vi "Arduino-Open.vi"(6 "Max number timeouts":u32=20, 7 "Enable Termination\nChar (T)":bool=TRUE, 8 "error in (no error)":errorcluster, 9 "termination char\n(0xA = '\\n' = LF)":u8=10 format="%.0x", 10 "baud rate (9600)":u32=9600, 11 "Visa Resource":refnum<visa-resource-name>) -> (0 "error out":errorcluster, 2 "Moin, moin!":string, 3 "VISA resource name out":refnum<visa-resource-name>)   [LabVIEW 2018]
uses:
  <vilib>/Instr/_visa.llb/VISA Configure Serial Port (Instr).vi
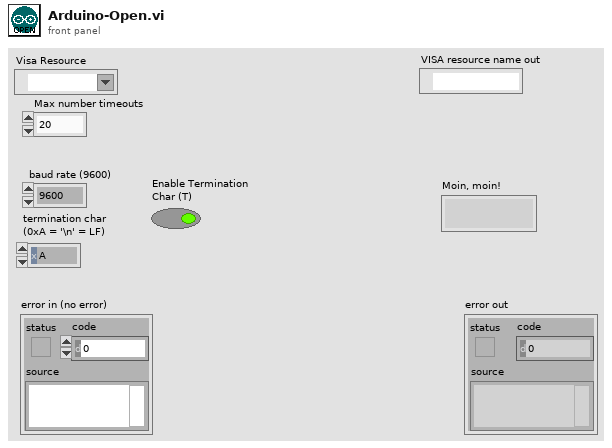
[diagram p1: front panel]
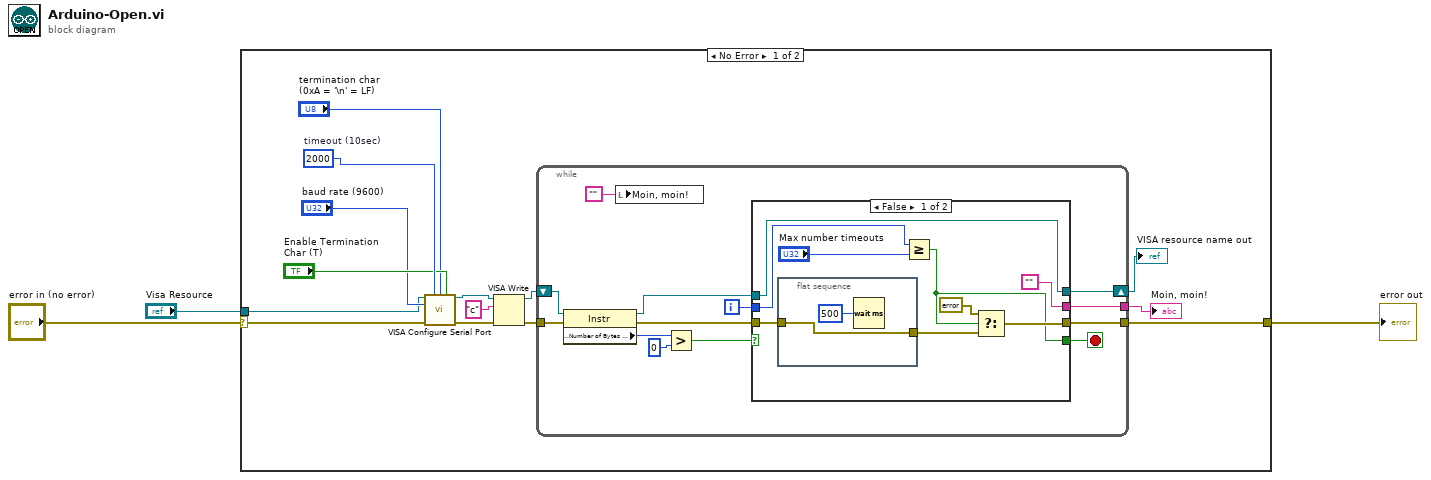
[diagram p0: block diagram]
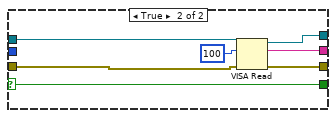
[diagram p2: hidden frame]
diagram:
  n1 = case shown="No Error" "error in (no error)" {
    selector: "error in (no error)" -> [w6 w49]
    tunnel: [w7 w49] -> w3
    tunnel: "Visa Resource" -> [w5 _]
    frame No Error {
      w14 = u32 2000  # timeout (10sec)
      n2 = call-poly "VISA Configure Serial Port"("VISA resource name"=w5, "timeout (10sec)"=w14, "termination char\n(0xA = '\\n' = LF)"="termination char\n(0xA = '\\n' = LF)", "Enable Termination\nChar (T)"="Enable Termination\nChar (T)", "baud rate (9600)"="baud rate (9600)", "error in (no error)"=w6) -> ("VISA resource name out"=w13:refnum<visa-resource-name>, "error out"=w12:errorcluster)  [unwired: 8 in]
      n3 = VISA Write(VISA resource name=w13, write buffer="c", error in (no error)=w12) -> (VISA resource name out=w15:refnum<visa-resource-name>, error out=w17:errorcluster)  [unwired: 1 out]
      n4 = while {
        shift-right: [w25] -> w4
        shift-left: w15 -> [w28]
        tunnel: [w24] -> w7
        tunnel: [w23] -> w16
        tunnel: w17 -> [w22]
        i -> [w18]
        stop <- w19 stop-if-true
        n5 = property class="Instr"(reference=w28, error in=w22) -> (reference out=w27:refnum<visa-resource-name>, error out=w21:errorcluster, "Serial Settings:Number of Bytes at Serial Port"=w30:u32)
        n6 = local write "Moin, moin!"("") -> ()
        n7 = Greater?(x=w30, y=0) -> (0:w26:bool)
        n8 = case shown="False" w26 {
          selector: w26 -> [_ w42]
          tunnel: w27 -> [w32 w48]
          tunnel: [w32 w47] -> w25
          tunnel: [w35 w46] -> w24
          tunnel: ["" w45] -> w23
          tunnel: w21 -> [w31 w44]
          tunnel: [w34 w42] -> w19
          tunnel: w18 -> [w37 _]
          frame False {
            n9 = flat-sequence {
              tunnel: [w40] -> w33
              tunnel: w31 -> [w40]
              frame #0 {
                n10 = Wait (ms)(milliseconds to wait=u32 500) -> ()  [unwired: 1 out]
              }
            }
            n11 = Greater Or Equal?(x=w37, y="Max number timeouts") -> (x >= y?=w34:bool)
            n12 = Select(t=errorcluster {"status"=TRUE, "code"=5002, "source"="Init.vi.  Unable to establish connection with Arduino.  Please ensure that you have selected the correct COM port and that you have flashed the Arduino with the correct firmware."} ("error out"), s=w34, f=w33) -> (s? t:f=w35:errorcluster)
          }
          frame True {
            n13 = VISA Read(VISA resource name=w48, byte count=100, error in (no error)=w44) -> (VISA resource name out=w47:refnum<visa-resource-name>, read buffer=w45:string, error out=w46:errorcluster)  [unwired: 1 out]
          }
        }
      }
      "Moin, moin!" <- w16
      "VISA resource name out" <- w4
    }
    frame Error {
    }
  }
  "error out" <- w3
